vi "dummy.read.ccd.vi"() -> (3 "Array":i32[](array[numeric]))   [LabVIEW 2022 SP3]
uses:
  <vilib>/Analysis/NI_AALBase.lvlib
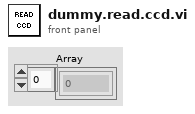
[diagram p1: front panel]
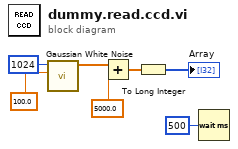
[diagram p0: block diagram]
diagram:
  n1 = call <vilib>:"Gaussian White Noise.vi"("standard deviation"=100.0, "samples"=1024) -> ("Gaussian noise pattern"=w3:dbl[])  [unwired: 8 in, 1 out]
  n2 = Add(x=w3, y=5000.0) -> (x+y=w6:dbl[])
  n3 = To Long Integer(number=w6) -> (32bit integer=→"Array":i32[])
  n4 = Wait (ms)(milliseconds to wait=u32 500) -> ()  [unwired: 1 out]
